vi "StopSTSmouse.vi"(8 "error in (no error)":errorcluster, 11 "Application ref in":refnum<vi>) -> (0 "error out":errorcluster, 3 "Application ref out":refnum<vi>)   [LabVIEW 2014]
uses:
  <userlib>/Nanonis Prog Interface V5/Nanonis Prog Interface.lvlib
panel:
  in  "nMilliseconds":i32=2000
  in  "AutoItX3Lib.IAutoItX3":refnum<k7>
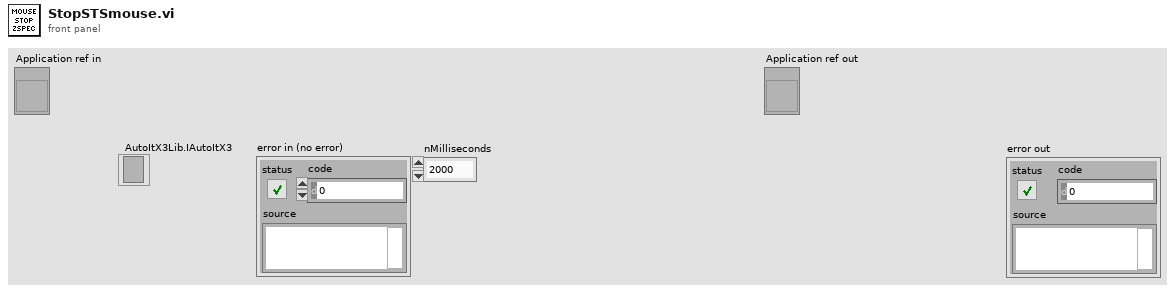
[diagram p1: front panel]
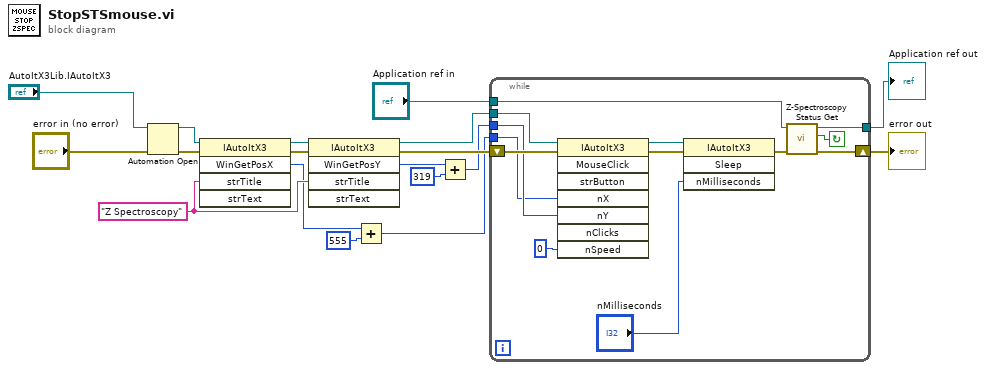
[diagram p0: block diagram]
diagram:
  w12 = "Z Spectroscopy" ("strTitle")
  n1 = Automation Open(error in (no error)="error in (no error)", Automation Refnum="AutoItX3Lib.IAutoItX3") -> (Automation Refnum=w14:refnum<k7>, error out=w15:errorcluster)  [unwired: 2 in]
  n2 = invoke class="IAutoItX3" method="WinGetPosX"(reference=w14, error in=w15, "strTitle"=w12) -> (reference out=w10:refnum<k7>, error out=w11:errorcluster, "WinGetPosX"=w8:i32)  [unwired: 2 in, 2 out]
  n3 = invoke class="IAutoItX3" method="WinGetPosY"(reference=w10, error in=w11, "strTitle"=w12) -> (reference out=w17:refnum<k7>, error out=w16:errorcluster, "WinGetPosY"=w9:i32)  [unwired: 2 in, 2 out]
  n4 = Add(x=w8, y=555) -> (x+y=w5:i32)
  n5 = Add(x=w9, y=319) -> (x+y=w7:i32)
  n6 = while {
    tunnel: w17 -> [w31]
    tunnel: w7 -> [w29]
    tunnel: w5 -> [w26]
    shift-right: [w21] -> w3
    shift-left: w16 -> [w30]
    tunnel: "Application ref in" -> [w20]
    tunnel: [w19] -> w1
    stop <- w23 continue-if-true
    n7 = invoke class="IAutoItX3" method="MouseClick"(reference=w31, error in=w30, "nX"=w26, "nY"=w29, "nSpeed"=0) -> (reference out=w28:refnum<k7>, error out=w27:errorcluster)  [unwired: 3 in, 6 out]
    n8 = invoke class="IAutoItX3" method="Sleep"(reference=w28, error in=w27, "nMilliseconds"="nMilliseconds") -> (error out=w22:errorcluster)  [unwired: 1 in, 3 out]
    n9 = call <userlib>:"Z-Spectroscopy Status Get.vi"("Error in (no error)"=w22, "Application ref in"=w20) -> ("Error out"=w21:errorcluster, "Running?"=w23:bool, "Application ref out"=w19:refnum<vi>)  [unwired: 5 in]
  }
  "error out" <- w3
  "Application ref out" <- w1
